vi "Write GISPollStatus.vi"(7 "ForceEvent":bool, 8 "error in (no error)":errorcluster, 10 "GISHeadStatus":T1[](array[typedef]), 11 "GIS Printer in":refnum<class "GIS Printer.lvclass">) -> (0 "error out":errorcluster, 3 "GIS Printer out":refnum<class "GIS Printer.lvclass">)   [LabVIEW 2022 SP3, in "GIS Printer.lvclass"]
uses:
  GIS Printer.lvclass
  Typedefs/GIS Status--Cluster.ctl
  GIS Printer.lvclass/GIS Printer.ctl
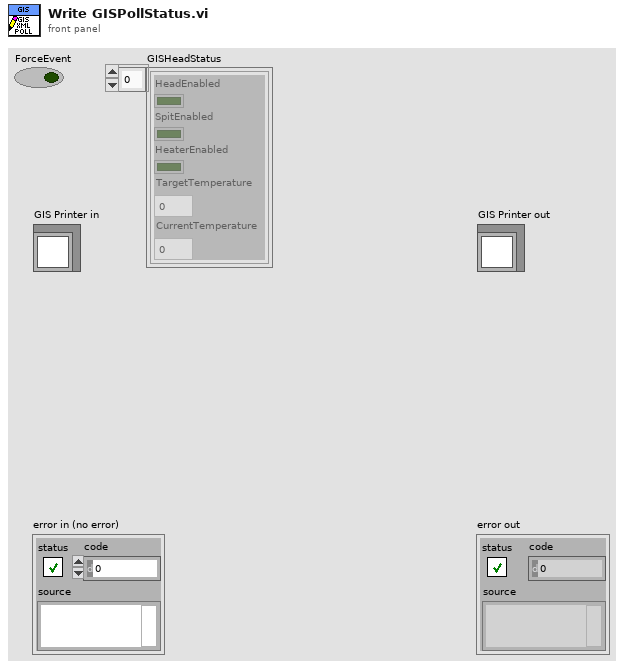
[diagram p1: front panel]
types:
  T1 = typedef "GIS Status--Cluster.ctl" = cluster{"HeadEnabled":bool, "SpitEnabled":bool, "HeaterEnabled":bool, "TargetTemperature":dbl, "CurrentTemperature":dbl}
  T2 = typedef "GIS Printer.lvclass/Private Data.ctl" = cluster{"UserEvents":T3, "All Dependencies":cluster{"Class References":refnum<class>[], "Class Names":string[]}, "PrinterConiguration":T4, "Status":T5, "GISHeadStatus":T1[], "HeadStatus":T6}
  T3 = typedef "GIS Printer.lvclass/UserEvents.ctl" = cluster{"API Incoming Event":refnum<user-event>, "API Executed Event":refnum<user-event>, "API Return Event":refnum<user-event>, "Status Changed Event":refnum<user-event>, "Abort":refnum<user-event>, "stop process":refnum<user-event>, "GISPollStatus":refnum<user-event>, "GISHeadStatus":refnum<user-event>, "Error Event":refnum<user-event>}
  T4 = typedef "GIS Printer.lvclass/PrinterConfiguration--Cluster.ctl" = cluster{"IPAddress":string, "Move Stage on RTP Command?":bool, "Stage Move Position":string, "PH1-Prime Path":path, "PH2-Prime Path":path, "PH3-Prime Path":path, "PH4-Prime Path":path, "PH5-Prime Path":path, "PH6-Prime Path":path, "PrintScriptsFolder":path, "PurgeScriptsFolder":path, "StageScriptsFolder":path, "PH1-HeatOn Path":path, "PH2-HeatOn Path":path, "PH3-HeatOn Path":path, "PH4-HeatOn Path":path, "PH5-HeatOn Path":path, "PH6-HeatOn Path":path, "PH1-HeatOff Path":path, "PH2-HeatOff Path":path, "PH3-HeatOff Path":path, "PH4-HeatOff Path":path, "PH5-HeatOff Path":path, "PH6-HeatOff Path":path}
  T5 = typedef "GIS Printer.lvclass/Status Cluster.ctl" = cluster{"Command Status":variant, "TCP Commands & Responses":string[][], "Printer Busy?":bool}
  T6 = typedef "HeadEnableStatus--cluster.ctl" = cluster{"PH1_Enable":bool, "PH2_Enable":bool, "PH3_Enable":bool, "PH4_Enable":bool, "PH5_Enable":bool, "PH6_Enable":bool}
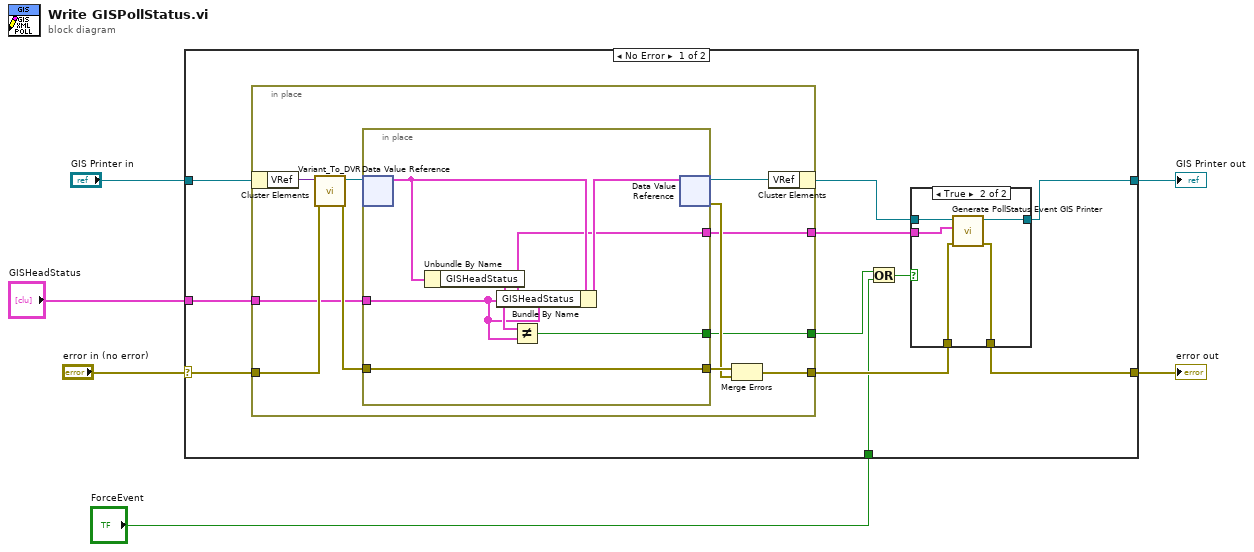
[diagram p0: block diagram]
diagram:
  n1 = case shown="No Error" "error in (no error)" {
    selector: "error in (no error)" -> [w16 w42]
    tunnel: [w10 w42] -> w5
    tunnel: [w12 w43] -> w3
    tunnel: "GIS Printer in" -> [w17 w43]
    tunnel: "GISHeadStatus" -> [w15 _]
    tunnel: "ForceEvent" -> [w7 _]
    frame No Error {
      n2 = in-place {
        in-place-border: w16 -> [w33]
        in-place-border: [w29] -> w11
        in-place-border: w15 -> [w27]
        in-place-border: [w26] -> w14
        in-place-border: [w25] -> w9
        n3 = in-place-cluster #1(w17) -> ("VRef"=w35:variant)
        n4 = call "Variant_To_DVR.vi"("error in (no error)"=w33, "Variant"=w35) -> ("error out"=w32:errorcluster, "DVR"=w34:refnum<data-value>)  [unwired: 8 in]
        n5 = in-place {
          in-place-border: w32 -> [w41]
          in-place-border: [w41] -> w31
          in-place-border: w27 -> [w36]
          in-place-border: [w37] -> w26
          in-place-border: [w36] -> w25
          n6 = in-place-dvr #2(w34) -> (w39:T2)  [unwired: 1 out]
          n7 = Unbundle By Name(w39) -> ("GISHeadStatus"=w38:T1[])
          n8 = Bundle By Name(cluster=w39, "GISHeadStatus"=w36) -> (w40:T2)
          n9 = Not Equal?(x=w38, y=w36) -> (x != y?=w37:bool)
          n10 = in-place-dvr #2(w40) -> (w28:refnum<data-value>, w30:errorcluster)
        }
        n11 = Merge Errors(w31, w30) -> (w29:errorcluster)
        n12 = in-place-cluster #1("VRef"=w28) -> (w13:refnum<class "GIS Printer.lvclass">)
      }
      n13 = Or(x=w14, y=w7) -> (x .or. y?=w8:bool)
      n14 = case shown="True" w8 {
        tunnel: w13 -> [w19 w24]
        tunnel: [w19 w23] -> w12
        tunnel: w11 -> [w18 w22]
        tunnel: [w18 w21] -> w10
        tunnel: w9 -> [_ w20]
        frame False {
        }
        frame True {
          n15 = call "Generate PollStatus Event GIS Printer.vi"("error in (no error)"=w22, "GISHeadStatus"=w20, "GIS Printer in"=w24) -> ("error out"=w21:errorcluster, "GIS Printer out"=w23:refnum<class "GIS Printer.lvclass">)  [unwired: 7 in]
        }
      }
    }
    frame Error {
    }
  }
  "error out" <- w5
  "GIS Printer out" <- w3
